vi "Set Simulation mode.vi"(8 "error in (no error)":errorcluster, 11 "Simulation mode (T)":bool=TRUE) -> (0 "error out (passthrough)":errorcluster)   [LabVIEW 2019, in "ACSVcontrol-driver.lvlib"]
doc: "If input is true, sets the driver into a Simulation mode. Instead of sending the packets, the driver will do nothing and will simulate the device as it would have been working and connected."
uses:
  ACSVcontrol-driver.lvlib
  Private/Globals.vi
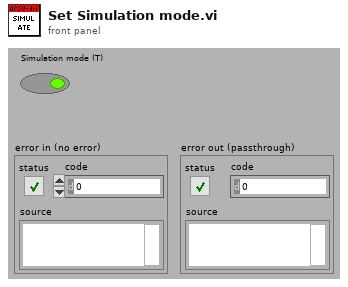
[diagram p1: front panel]
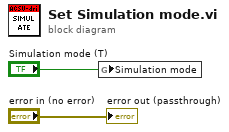
[diagram p0: block diagram]
diagram:
  n1 = global write "Globals.vi" "Simulation mode"("Simulation mode (T)") -> ()
  "error out (passthrough)" <- "error in (no error)"
